vi "JVS PJVS GUI Main.vi"() -> ()   [LabVIEW 2020]
uses:
  External control/DataSocketCluster external.ctl
  <instrlib>/niFgen/niFgen.llb/niFgen_ctl Sample Clock Source Values (Ring).ctl
panel:
  out "Array":T1(array[cluster]) {"Segment Q state" min=-1 max=1 step=1 scale=-1.0..1.0}
  out "actual FGEN handle":refnum<k15> caption="Instrument Handle Out"
  in  "?":T2(tab)
  in  "Compensate f for Ext clock":bool=TRUE caption="Compensate frequency for Ext clock?"
  in  "Set Trig out Frame/Update":bool caption="Set Trig out"
  in  "Set Ext clock on/off":bool caption="Set Ext clock"
  in  "Set AC wave":bool
  in  "PJVS steps":u32=100
  in  "Frequency (Hz)":dbl=100.0 format="%#_10g"
  in  "Send AC sine":bool
  in  "Send DC string":bool
  in  "DC-String":string="SETDC_MMMMMMMMMMOO"
  in  "Send 0 V to bias source":bool
  in  "Amplitude (V)":dbl=1.0
  in  "0: sine, 1: triang":bool
  out "Calculated time on PJVS step\n(smallest value is 17)":u32=100
  out "Return time interval on PJVS step":string
  out "PJVS steps for AC waveform":dbl[](graph)
  out "Voltage at each step on PJVS curve":dbl[](array[numeric]) format="%#_16g"
  in  "Stop trigger":bool caption="Stop"
  in  "Amplitude":dbl=2.0 format="%0_3g"
  in  "Frequency":dbl=1000000.0 format="%.2p"
  in  "Standard Waveform":u16(ring) items=["Sine", "Square", "Triangle", "Ramp Up", "Ramp Down", "DC", "Noise"]
  in  "FGEN Resource Name":refnum<k15>
  in  "Start trigger":bool
  in  "Channel":string="0"
  in  "Source (Onboard Clock)":T3="OnboardClock"
  in  "This machine (client)":string="localhost"
  in  "Name of computer":string="CZC105BD8M"
  in  "TimeOut Time (s)":dbl=5.0 format="%.2f"
  out "Response from NPL bias source":string
  out "error out":errorcluster {"code" format="%.0x"}
  out "machine":T4 {"TimeStamp" format="%.2f"}
  in  "Quit":bool
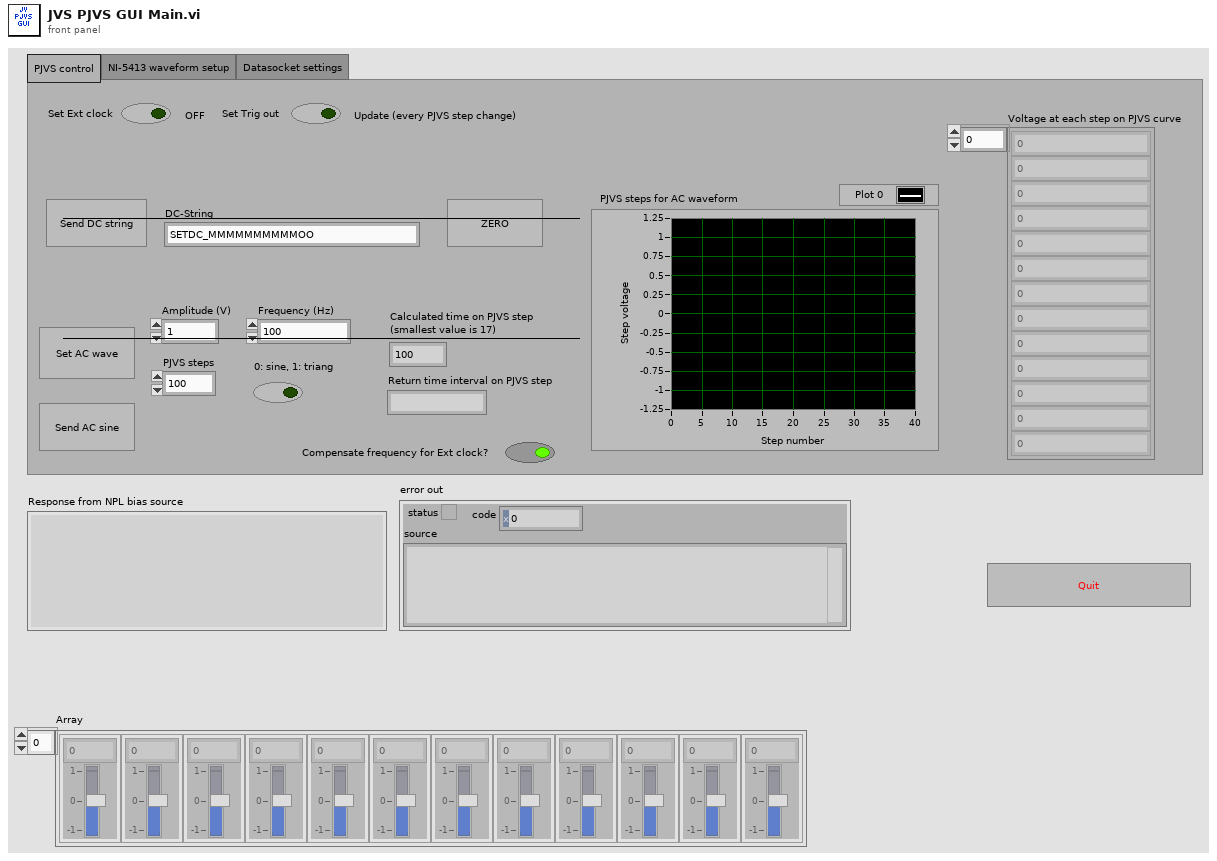
[diagram p1: front panel]
types:
  T1 = cluster{"Segment ID":dbl, "Segment Q state":i32}[]
  T2 = enum32{"PJVS control", "NI-5413 waveform setup", "Datasocket settings"}
  T3 = typedef "niFgen_ctl Sample Clock Source Values (Ring).ctl" = string
  T4 = typedef "DataSocketCluster external.ctl" = cluster{"Server Machine":string, "Client Machine":string, "Data":string, "TimeStamp":dbl, "Count":i32, "Target Process":string}
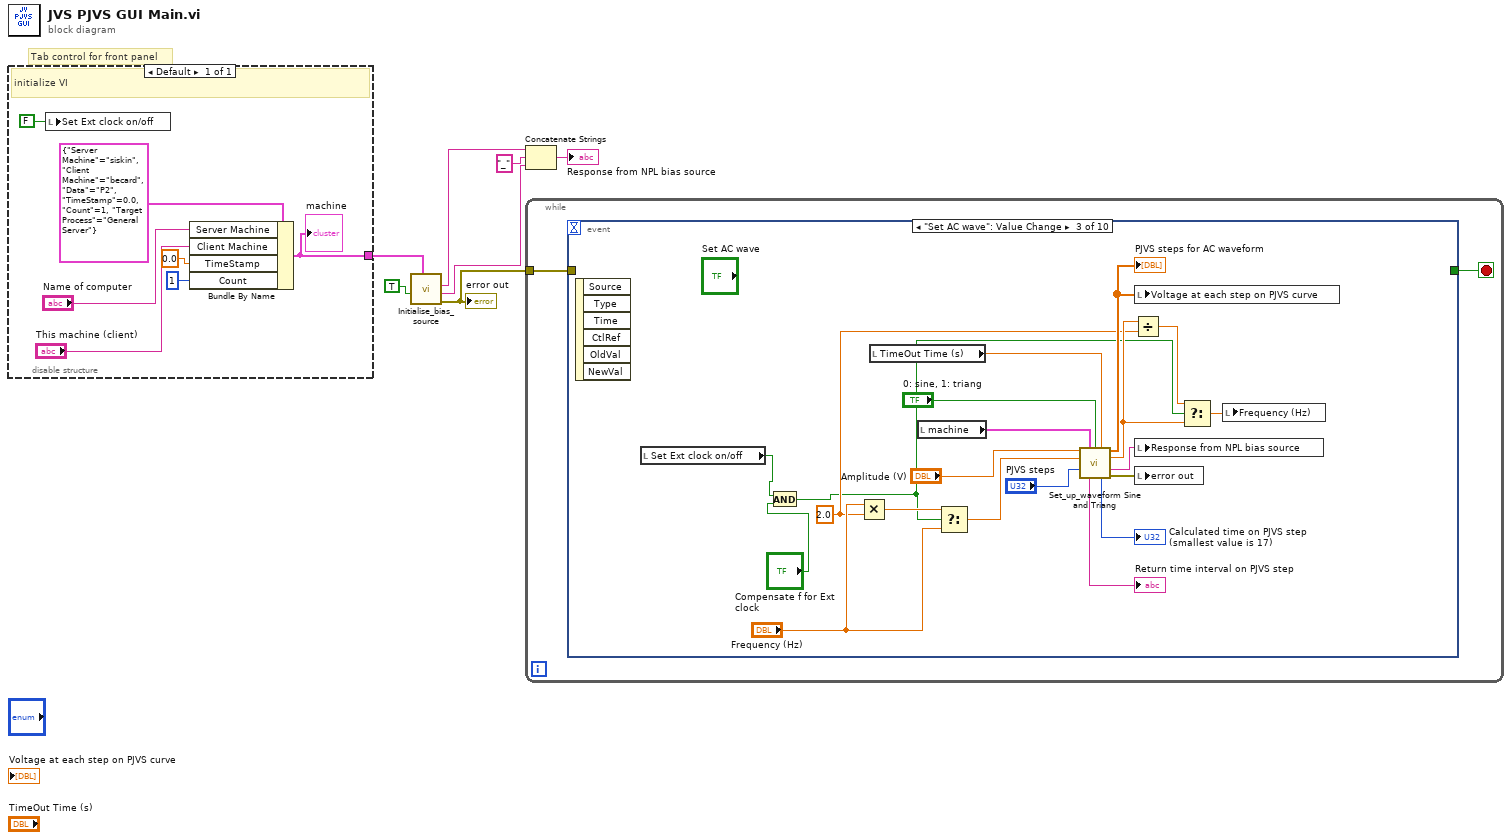
[diagram p0: block diagram]
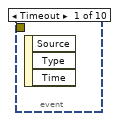
[diagram p2: hidden frame]
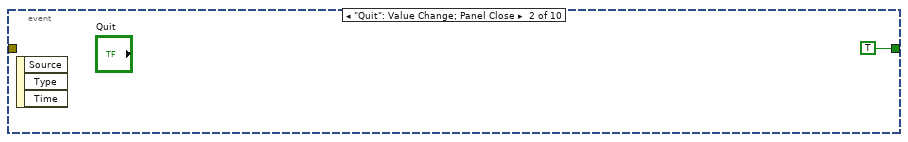
[diagram p3: hidden frame]
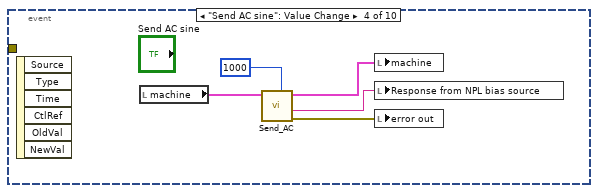
[diagram p4: hidden frame]
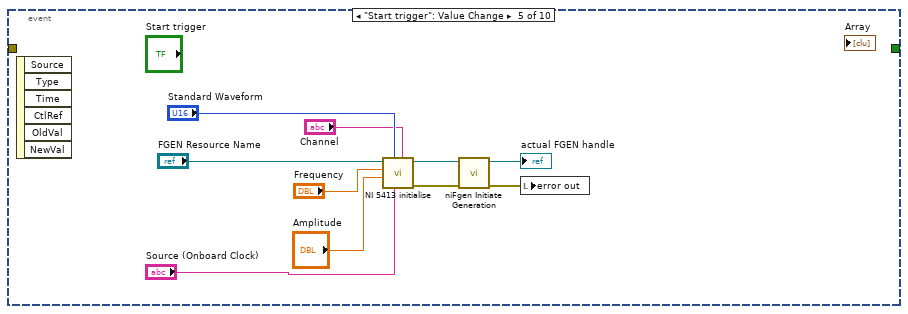
[diagram p5: hidden frame]
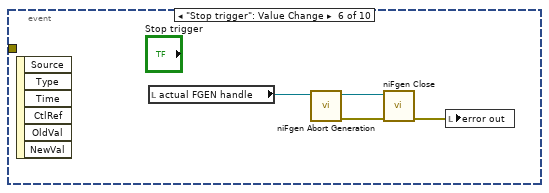
[diagram p6: hidden frame]
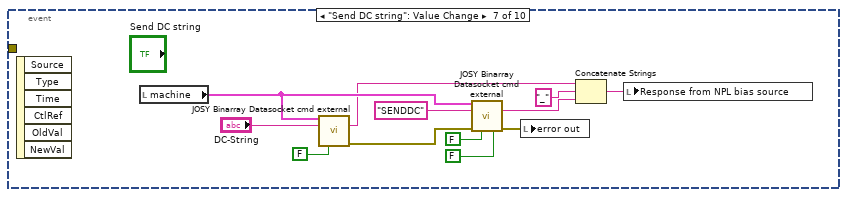
[diagram p7: hidden frame]
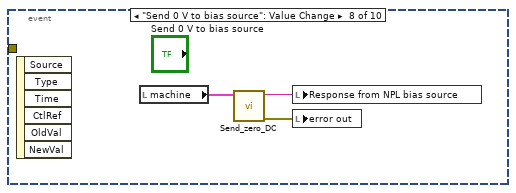
[diagram p8: hidden frame]
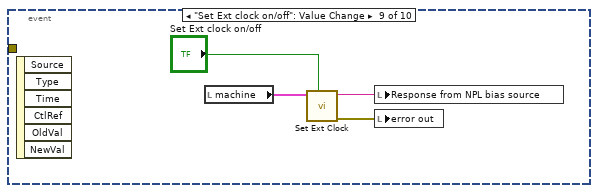
[diagram p9: hidden frame]
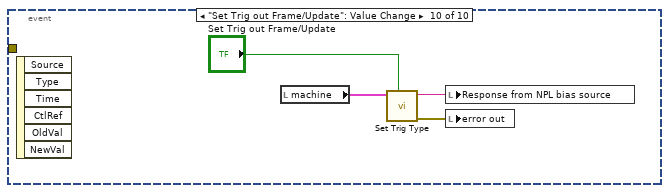
[diagram p10: hidden frame]
diagram:
  # "Tab control for front panel"
  n1 = disable-structure shown="Default" {
    disable-tunnel: [w9] -> w7
    frame Enabled {
      # "initialize VI"
      n2 = local write "Set Ext clock on/off"(FALSE ("Set Ext clock on/off")) -> ()
      n3 = Bundle By Name(cluster=T4 {"Server Machine"="siskin", "Client Machine"="becard", "Data"="P2", "TimeStamp"=0.0, "Count"=1, "Target Process"="General Server"} ("DataSocketCluster In"), "Server Machine"="Name of computer", "Client Machine"="This machine (client)", "TimeStamp"=0.0, "Count"=1) -> (w9:T4)
      "machine" <- w9
    }
  }
  n4 = call "Initialise_bias_source.vi"("output cluster"=w7, "Load bias parameters"=TRUE) -> ("error out"=w6:errorcluster, "Response to Load bias parameters"=w4:string, "Response Initialise"=w2:string)  [unwired: 7 in]
  "error out" <- w6
  n5 = Concatenate Strings(w2, "_" ("string"), w4) -> (→"Response from NPL bias source":string)
  n6 = while {
    tunnel: w6 -> [w15]
    stop <- w16 stop-if-true
    n7 = event shown="[2] \"Set AC wave\": Value Change" {
      selector: _ -> [_ _ _ _ _ _ _ _ _ _]
      dyn-events: _ -> [_ _ _ _ _ _ _ _ _ _]
      timeout: _ -> [_ _ _ _ _ _ _ _ _ _]
      tunnel: [_ TRUE _ _ _ _ _ _ _ _] -> w16
      tunnel: w15 -> [_ _ _ _ _ _ _ _ _ _]
      event Timeout {
        n8 = event-data() -> ()  [unwired: 1 in, 3 out]
      }
      event "Quit": Value Change; Panel Close {
        n9 = event-data() -> ()  [unwired: 1 in, 3 out]
      }
      event "Set AC wave": Value Change {
        w21 = 2.0 ("y")
        n10 = event-data() -> ()  [unwired: 1 in, 6 out]
        n11 = local read "Set Ext clock on/off"() -> (w19:bool)
        n12 = And(x=w19, y="Compensate f for Ext clock") -> (x .and. y?=w18:bool)
        n13 = Multiply(x="Frequency (Hz)", y=w21) -> (x*y=w26:dbl)
        n14 = local read "TimeOut Time (s)"() -> (w33:dbl)
        n15 = local read "machine"() -> (w32:T4)
        n16 = Select(t=w26, s=w18, f="Frequency (Hz)") -> (s? t:f=w25:dbl)
        n17 = call "Set_up_waveform Sine and Triang.vi"("Amplitude (V)"="Amplitude (V)", "DataSocketCluster In"=w32, "0: sine, 1: triang"="0: sine, 1: triang", "TimeOut Time (s)"=w33, "Frequency (Hz)"=w25, "Steps on PJVS curve"="PJVS steps") -> ("Voltage at each step on PJVS curve"=w28:dbl[], "Set frequency (Hz)"=w22:dbl, "Returned number of steps on PJVS curve"=w34:string, "Returned time interval on each step"=→"Return time interval on PJVS step":string, "Calculated time on step (smallest value is 17)"=→"Calculated time on PJVS step\n(smallest value is 17)":u32, "error IO"=w37:errorcluster)  [unwired: 4 in]
        "PJVS steps for AC waveform" <- w28
        n18 = Divide(x=w22, y=w21) -> (x/y=w24:dbl)
        n19 = local write "Voltage at each step on PJVS curve"(w28) -> ()
        n20 = local write "Response from NPL bias source"(w34) -> ()
        n21 = local write "error out"(w37) -> ()
        n22 = Select(t=w24, s=w18, f=w22) -> (s? t:f=w23:dbl)
        n23 = local write "Frequency (Hz)"(w23) -> ()
      }
      event "Send AC sine": Value Change {
        n24 = event-data() -> ()  [unwired: 1 in, 6 out]
        n25 = local read "machine"() -> (w39:T4)
        n26 = call "Send_AC.vi"("milliseconds to wait"=u32 1000, "DataSocketCluster In"=w39) -> ("error out"=w41:errorcluster, "Response to SEND AC"=w40:string, "DataSocketCluster out"=w38:T4)  [unwired: 7 in]
        n27 = local write "machine"(w38) -> ()
        n28 = local write "Response from NPL bias source"(w40) -> ()
        n29 = local write "error out"(w41) -> ()
      }
      event "Start trigger": Value Change {
        n30 = event-data() -> ()  [unwired: 1 in, 6 out]
        n31 = call "NI 5413 initialise.vi"("Channel"="Channel", "Source (Onboard Clock)"="Source (Onboard Clock)", "Standard Waveform"="Standard Waveform", "Amplitude"="Amplitude", "Frequency"="Frequency", "FGEN Resource Name"="FGEN Resource Name") -> ("error out"=w46:errorcluster, "Instrument Handle Out"=w44:refnum<k15>)  [unwired: 4 in]
        n32 = call <instrlib>:"niFgen Initiate Generation.vi"("error in (no error)"=w46, "Instrument Handle"=w44) -> ("error out"=w45:errorcluster, "Instrument Handle Out"=→"actual FGEN handle":refnum<k15>)  [unwired: 8 in]
        n33 = local write "error out"(w45) -> ()
      }
      event "Stop trigger": Value Change {
        n34 = event-data() -> ()  [unwired: 1 in, 6 out]
        n35 = local read "actual FGEN handle"() -> (w54:refnum<k15>)
        n36 = call <instrlib>:"niFgen Abort Generation.vi"("Instrument Handle"=w54) -> ("error out"=w56:errorcluster, "Instrument Handle Out"=w55:refnum<k15>)  [unwired: 9 in]
        n37 = call <instrlib>:"niFgen Close.vi"("error in (no error)"=w56, "Instrument Handle"=w55) -> ("error out"=w53:errorcluster)  [unwired: 9 in]
        n38 = local write "error out"(w53) -> ()
      }
      event "Send DC string": Value Change {
        n39 = event-data() -> ()  [unwired: 1 in, 6 out]
        n40 = local read "machine"() -> (w65:T4)
        n41 = call "JOSY Binarray Datasocket cmd external.vi"("DataSocketCluster In"=w65, "Command"="DC-String", "Command has variable"=FALSE) -> ("Reply data"=w57:string, "error out"=w66:errorcluster)  [unwired: 9 in, 2 out]
        n42 = call "JOSY Binarray Datasocket cmd external.vi"("DataSocketCluster In"=w65, "Command"="SENDDC", "error in (no error)"=w66, "Command has variable"=FALSE, "String"=FALSE) -> ("Reply data"=w59:string, "error out"=w64:errorcluster)  [unwired: 7 in, 2 out]
        n43 = local write "error out"(w64) -> ()
        n44 = Concatenate Strings(w57, "_" ("string"), w59) -> (w58:string)
        n45 = local write "Response from NPL bias source"(w58) -> ()
      }
      event "Send 0 V to bias source": Value Change {
        n46 = event-data() -> ()  [unwired: 1 in, 6 out]
        n47 = local read "machine"() -> (w71:T4)
        n48 = call "Send_zero_DC.vi"("machine"=w71) -> ("error out"=w69:errorcluster, "String"=w70:string)  [unwired: 9 in]
        n49 = local write "Response from NPL bias source"(w70) -> ()
        n50 = local write "error out"(w69) -> ()
      }
      event "Set Ext clock on/off": Value Change {
        n51 = event-data() -> ()  [unwired: 1 in, 6 out]
        n52 = local read "machine"() -> (w73:T4)
        n53 = call "Set Ext Clock.vi"("Requested state of Ext clock"="Set Ext clock on/off", "machine"=w73) -> ("error out"=w74:errorcluster, "Reply data"=w75:string)  [unwired: 8 in]
        n54 = local write "Response from NPL bias source"(w75) -> ()
        n55 = local write "error out"(w74) -> ()
      }
      event "Set Trig out Frame/Update": Value Change {
        n56 = event-data() -> ()  [unwired: 1 in, 6 out]
        n57 = local read "machine"() -> (w79:T4)
        n58 = call "Set Trig Type.vi"("Requested state of Trig (off: Update)"="Set Trig out Frame/Update", "machine"=w79) -> ("error out"=w76:errorcluster, "Reply data"=w77:string)  [unwired: 8 in]
        n59 = local write "Response from NPL bias source"(w77) -> ()
        n60 = local write "error out"(w76) -> ()
      }
    }
  }
